vi "Write cookBehavior.vi"(8 "error in (no error)":errorcluster, 10 "cookBehavior":refnum<class "CookBehavior.lvclass">, 11 "Appliance in":refnum<class "Appliance.lvclass">) -> (0 "error out":errorcluster, 3 "Appliance out":refnum<class "Appliance.lvclass">)   [LabVIEW 2010, in "Appliance.lvclass"]
uses:
  Appliance.lvclass
  CookBehavior/CookBehavior.lvclass
  Appliance.lvclass/Appliance.ctl
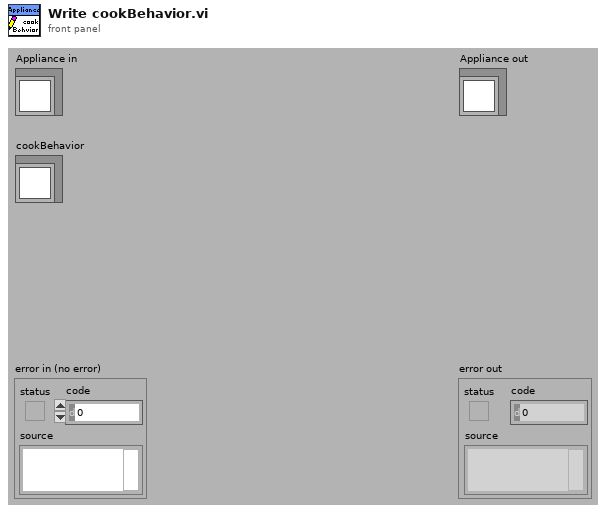
[diagram p1: front panel]
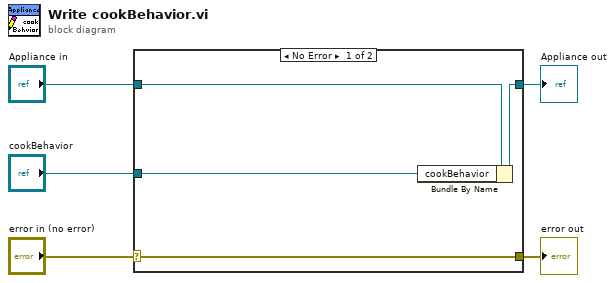
[diagram p0: block diagram]
diagram:
  n1 = case shown="No Error" "error in (no error)" {
    selector: "error in (no error)" -> [w9 w10]
    tunnel: [w9 w10] -> w4
    tunnel: [w7 w11] -> w2
    tunnel: "Appliance in" -> [w8 w11]
    tunnel: "cookBehavior" -> [w6 _]
    frame No Error {
      n2 = Bundle By Name(cluster=w8, "cookBehavior"=w6) -> (w7:refnum<class "Appliance.lvclass">)
    }
    frame Error {
    }
  }
  "error out" <- w4
  "Appliance out" <- w2
